vi "停止流程.vi"   [LabVIEW 2016]
types:
  T1 = cluster{"命令":string, cluster{"starting address":u16, "holding register value":u16}}
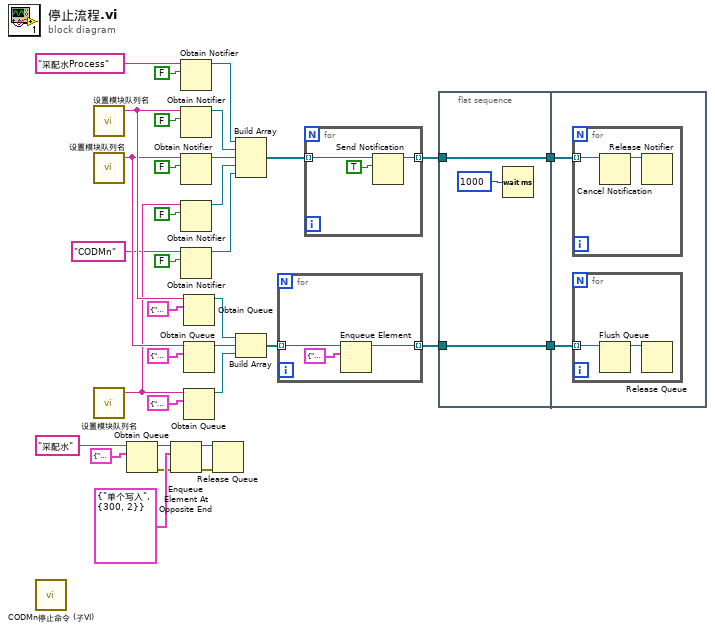
[diagram p0: block diagram]
diagram:
  n1 = call "CODMn停止命令 (子VI).vi"() -> ()  [unwired: 12 in]
  n2 = call "设置模块队列名.vi"() -> ("Msg"=w26:string)  [unwired: 5 in]
  n3 = call "设置模块队列名.vi"() -> ("Msg"=w23:string)  [unwired: 5 in]
  n4 = call "设置模块队列名.vi"() -> ("Msg"=w20:string)  [unwired: 5 in]
  n5 = Obtain Queue(name (unnamed)="采配水" ("名称（未命名）"), element data type=cluster{"命令":string, "数据":variant} {"命令"="", "数据"=variant}) -> (queue out=w29:refnum<queue>, error out=w2:errorcluster)  [unwired: 3 in, 1 out]
  n6 = Enqueue Element At Opposite End(queue=w29, element=T1 {"命令"="单个写入", {"starting address"=300, "holding register value"=2}} ("元素"), error in (no error)=w2) -> (queue out=w3:refnum<queue>, error out=w1:errorcluster)  [unwired: 1 in, 1 out]
  n7 = Obtain Notifier(name (unnamed)="采配水Process" ("名称（未命名）"), notification data type=FALSE) -> (notifier out=w17:refnum<notifier>)  [unwired: 2 in, 2 out]
  n8 = Obtain Notifier(name (unnamed)=w26, notification data type=FALSE) -> (notifier out=w16:refnum<notifier>)  [unwired: 2 in, 2 out]
  n9 = Obtain Notifier(name (unnamed)=w23, notification data type=FALSE) -> (notifier out=w15:refnum<notifier>)  [unwired: 2 in, 2 out]
  n10 = Obtain Notifier(name (unnamed)=w20, notification data type=FALSE) -> (notifier out=w14:refnum<notifier>)  [unwired: 2 in, 2 out]
  n11 = Obtain Notifier(name (unnamed)="CODMn" ("名称（未命名）"), notification data type=FALSE) -> (notifier out=w13:refnum<notifier>)  [unwired: 2 in, 2 out]
  n12 = Obtain Queue(name (unnamed)=w26, element data type=cluster{"命令":string, "data":variant} {"命令"="", "data"=variant}) -> (queue out=w12:refnum<queue>)  [unwired: 3 in, 2 out]
  n13 = Obtain Queue(name (unnamed)=w23, element data type=cluster{"命令":string, "data":variant} {"命令"="", "data"=variant}) -> (queue out=w11:refnum<queue>)  [unwired: 3 in, 2 out]
  n14 = Obtain Queue(name (unnamed)=w20, element data type=cluster{"命令":string, "data":variant} {"命令"="", "data"=variant}) -> (queue out=w10:refnum<queue>)  [unwired: 3 in, 2 out]
  n15 = Release Queue(queue=w3, error in (no error)=w1) -> ()  [unwired: 1 in, 3 out]
  n16 = Build Array(w17, w16, w15, w14, w13) -> (w8:refnum<notifier>[])
  n17 = Build Array(w12, w11, w10) -> (w9:refnum<queue>[])
  n18 = for {
    tunnel: w9 -> [w36] mode=indexing
    tunnel: [w35] -> w6 mode=indexing
    n19 = Enqueue Element(queue=w36, element=cluster{"命令":string, "data":variant} {"命令"="启动", "data"=variant(cluster{"站号":u16, "控制命令":u16[]} {"站号"=1, "控制命令"=[2816]})} ("启动命令")) -> (queue out=w35:refnum<queue>)  [unwired: 2 in, 2 out]
  }
  n20 = for {
    tunnel: w8 -> [w40] mode=indexing
    tunnel: [w38] -> w7 mode=indexing
    n21 = Send Notification(notification=TRUE ("通知"), notifier=w40) -> (notifier out=w38:refnum<notifier>)  [unwired: 1 in, 1 out]
  }
  n22 = flat-sequence {
    tunnel: w6 -> [w42]
    tunnel: w7 -> [w43]
    tunnel: [w43] -> w5
    tunnel: [w42] -> w4
    tunnel: w5 -> [w45]
    tunnel: w4 -> [w44]
    frame #0 {
      n23 = Wait (ms)(milliseconds to wait=u32 1000 ("等待时间（毫秒）")) -> ()  [unwired: 1 out]
    }
    frame #1 {
      n24 = for {
        tunnel: w45 -> [w49] mode=indexing
        n25 = Cancel Notification(0:w49) -> (8:w48:refnum<notifier>)  [unwired: 1 in, 2 out]
        n26 = Release Notifier(notifier=w48) -> ()  [unwired: 2 in, 3 out]
      }
      n27 = for {
        tunnel: w44 -> [w47] mode=indexing
        n28 = Flush Queue(queue=w47) -> (queue out=w46:refnum<queue>)  [unwired: 1 in, 2 out]
        n29 = Release Queue(queue=w46) -> ()  [unwired: 2 in, 3 out]
      }
    }
  }
